vi "Read High Cutoff Freq.vi"(8 "error in (no error)":errorcluster, 11 "DataFilter in":refnum<class "DataFilter.lvclass">) -> (0 "error out":errorcluster, 2 "High Cutoff Freq(Hz)":dbl, 3 "DataFilter out":refnum<class "DataFilter.lvclass">)   [LabVIEW 2010, in "DataFilter.lvclass"]
uses:
  DataFilter.lvclass
  DataFilter.lvclass/DataFilter.ctl
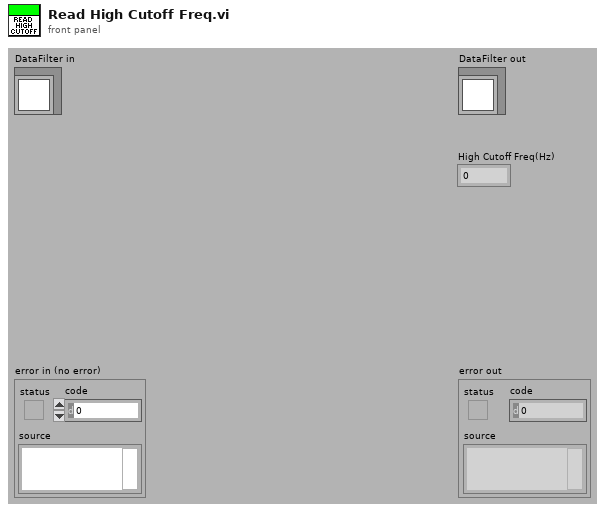
[diagram p1: front panel]
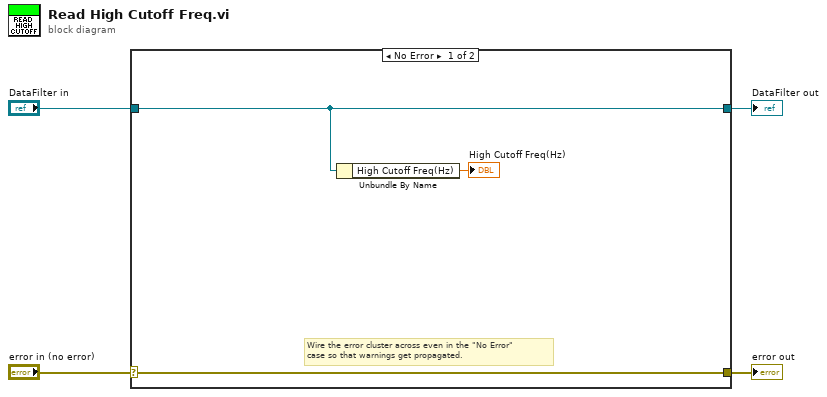
[diagram p0: block diagram]
diagram:
  n1 = case shown="No Error" "error in (no error)" {
    selector: "error in (no error)" -> [w7 w9]
    tunnel: [w7 w9] -> w3
    tunnel: [w6 w8] -> w1
    tunnel: "DataFilter in" -> [w6 w8]
    frame No Error {
      # "Wire the error cluster across even in the \"No Error\"\ncase so that warnings get propagated."
      n2 = Unbundle By Name(w6) -> ("High Cutoff Freq(Hz)"=→"High Cutoff Freq(Hz)":dbl)
    }
    frame Error {
    }
  }
  "error out" <- w3
  "DataFilter out" <- w1
